vi "CreateQueueNames.vi"(8 "error in (no error)":errorcluster, 10 "QueueNames":string[](array[string])=["QMH", "Class", "SP"], 11 "ModuleAdmin In":refnum<class "ModuleAdmin.lvclass">) -> (0 "error out":errorcluster, 2 "QueueNames Out":string[](array[string]), 3 "ModuleAdmin Out":refnum<class "ModuleAdmin.lvclass">)   [LabVIEW 2018, in "ScopePlugins.lvlib"]
doc: "This VI creates three individual queue names that can be used to create unique queues."
uses:
  ScopePlugins.lvlib
  <userlib>/NIST/ModuleAdminLib/ModuleAdmin/ModuleAdmin.lvclass
panel:
  out "QMH Queue Name":string
  out "Class Queue Name":string
  out "Measurement Acquisition  Loop Queue Name":string
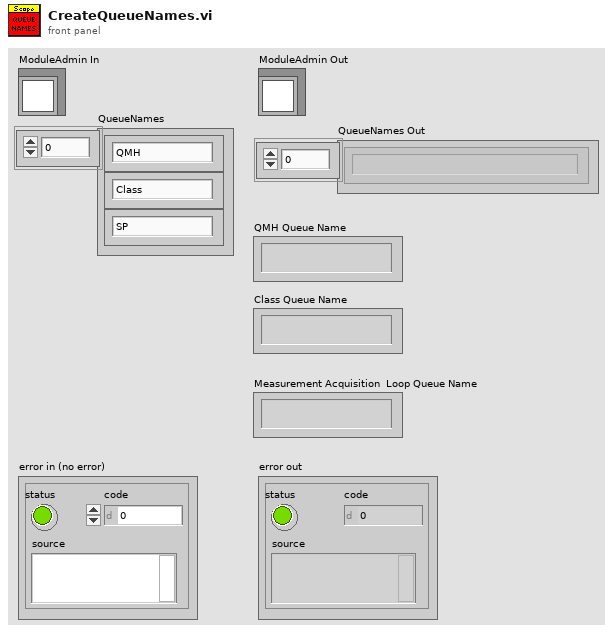
[diagram p1: front panel]
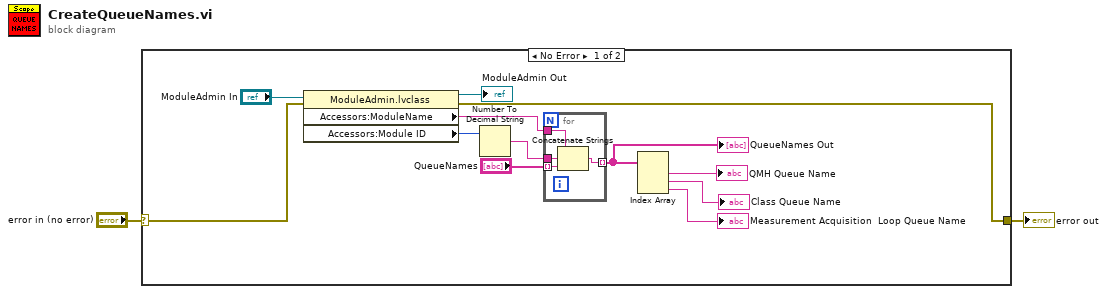
[diagram p0: block diagram]
diagram:
  n1 = case shown="No Error" "error in (no error)" {
    selector: "error in (no error)" -> [w9 w19]
    tunnel: [w8 w19] -> w2
    frame No Error {
      n2 = property class="ModuleAdmin.lvclass"(reference="ModuleAdmin In", error in=w9) -> (reference out=→"ModuleAdmin Out":refnum<class "ModuleAdmin.lvclass">, error out=w8:errorcluster, "Accessors:ModuleName"=w4:string, "Accessors:Module ID"=w5:i32)
      n3 = Number To Decimal String(number=w5) -> (decimal integer string=w6:string)  [unwired: 1 in]
      n4 = for {
        tunnel: [w18] -> w3 mode=indexing
        tunnel: w6 -> [w17]
        tunnel: "QueueNames" -> [w16] mode=indexing
        tunnel: w4 -> [w15]
        n5 = Concatenate Strings(w15, w17, w16) -> (w18:string)
      }
      "QueueNames Out" <- w3
      n6 = Index Array(array=w3) -> (element #1=→"QMH Queue Name":string, element #2=→"Class Queue Name":string, element #3=→"Measurement Acquisition  Loop Queue Name":string)  [unwired: 3 in]
    }
    frame Error {
    }
  }
  "error out" <- w2
